vi "Write View Data.vi"(8 "error in (no error)":errorcluster, 10 "View Data":variant, 11 "List Box View Model in":refnum<class "Control View Model.lvclass">) -> (0 "error out":errorcluster, 3 "List Box View Model out":refnum<class "Control View Model.lvclass">)   [LabVIEW 2020]
uses:
  Control View Model.lvclass
  Control View Model.lvclass/Control View Model.ctl
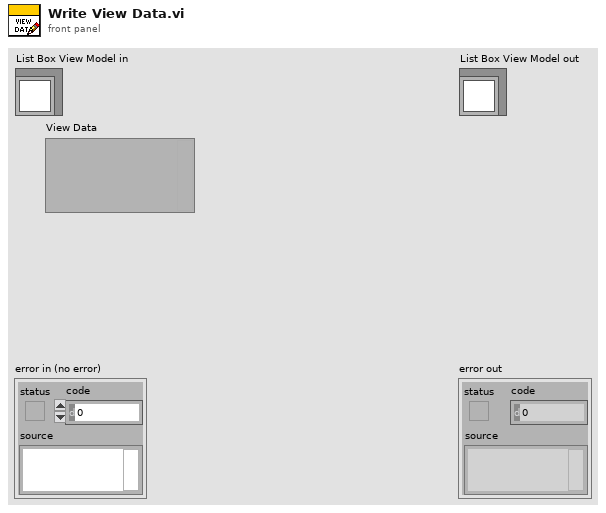
[diagram p1: front panel]
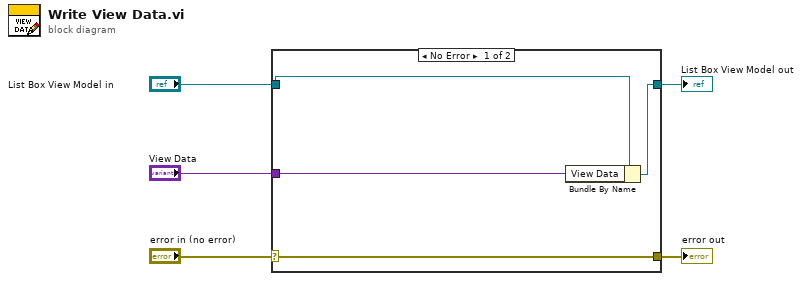
[diagram p0: block diagram]
diagram:
  n1 = case shown="No Error" "error in (no error)" {
    selector: "error in (no error)" -> [w9 w10]
    tunnel: [w9 w10] -> w4
    tunnel: [w7 w11] -> w2
    tunnel: "List Box View Model in" -> [w8 w11]
    tunnel: "View Data" -> [w6 _]
    frame No Error {
      n2 = Bundle By Name(cluster=w8, "View Data"=w6) -> (w7:refnum<class "Control View Model.lvclass">)
    }
    frame Error {
    }
  }
  "error out" <- w4
  "List Box View Model out" <- w2
